vi "Configure AO Channel.vi"(7 "instance":i32, 8 "error in":errorcluster, 10 "config":cluster{"carrier":dbl, "level":dbl}, 11 "lia host in":refnum<class "LIA Host Interface RT.lvclass">) -> (0 "error out":errorcluster, 3 "lia host out":refnum<class "LIA Host Interface RT.lvclass">)   [LabVIEW 2017, in "LIA Host Interface RT.lvclass"]
uses:
  LIA Host Interface RT.lvclass
  shared/Public/message.ctl
  shared/Lock-In Amplifier Example Shared.lvlib
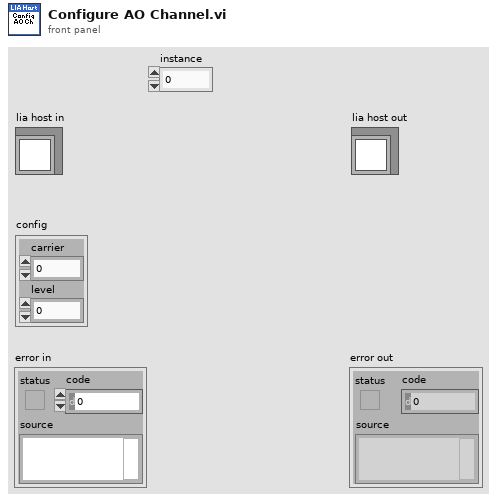
[diagram p1: front panel]
types:
  T1 = typedef "Lock-In Amplifier Example Shared.lvlib/message.ctl" = cluster{"command":u32, "payload":string}
  T2 = cluster{"instance":i32, "config":cluster{"carrier":dbl, "level":dbl}}
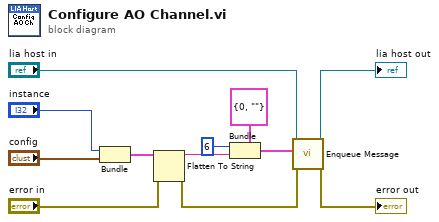
[diagram p0: block diagram]
diagram:
  n1 = Bundle("instance"="instance", "config"="config") -> (w10:T2)  [unwired: 1 in]
  n2 = Flatten To String(anything=w10, error in (no error)="error in") -> (data string=w8:string, error out=w5:errorcluster)  [unwired: 2 in, 1 out]
  n3 = Bundle(cluster=T1 {"command"=0, "payload"=""} ("message"), "command"=u32 6, "payload"=w8) -> (w7:T1)
  n4 = call "Enqueue Message.vi"("error in"=w5, "command"=w7, "lia host in"="lia host in") -> ("error out"=→"error out":errorcluster, "lia host out"=→"lia host out":refnum<class "LIA Host Interface RT.lvclass">)  [unwired: 7 in]
